vi "Line Configuration Dialog.vi"(8 "error in":errorcluster, 9 "engine configuration in":refnum<class "engine configuration.lvclass">, 10 "tag bus configurable plugin module configuration":refnum<class "Sequencer Module configuration.lvclass">, 11 "Line":T3) -> (0 "error out":errorcluster, 1 "success":bool, 2 "changed":bool, 3 "Mappings out":T2)   [LabVIEW 2015, in "Sequencer Module editor node.lvclass"]
doc: "A dialog for allowing a user to specify the values of a new line."
uses:
  Sequencer Module editor node.lvclass
  module/configuration/Line.ctl
  <vilib>/NI/Tag Bus Module Framework/channel/TBM channel.lvclass
  classes/Sequence/Config/Sequence Config.lvclass
  Mappings.ctl
  Map.ctl
  module/configuration/permissions.ctl
  <vilib>/NI/Module Execution Interface/Engine Configuration/engine configuration.lvclass
  module/configuration/Sequencer Module configuration.lvclass
  <vilib>/NI/Configuration Framework/serializable configuration/NISE_CEF_serializable configuration.lvclass/NISE_CEF_serializable configuration.ctl
  <vilib>/NI/Configuration Framework/serializable configuration/Read UID.vi
  <vilib>/Utility/LVClass/Get LV Class Name.vi
  <vilib>/NI/Configuration Framework/error generator/NISE_error generator.vi
  <vilib>/NI/Tag Bus/tag/tag descriptor.lvclass
  <vilib>/NI/DCAF UI Toolkit/Controls/DCAF UI Elements.lvlib
panel:
  out "errors":string
  in  "Access Type":T1
  in  "Tag":i32(listbox)
  in  "Data Type":i32(listbox)
  in  "Channel Name":string
  in  "cancel":bool
  in  "ok":bool
  # "#CodeRecommended Add implementation details here. For example, a shared variable URL."
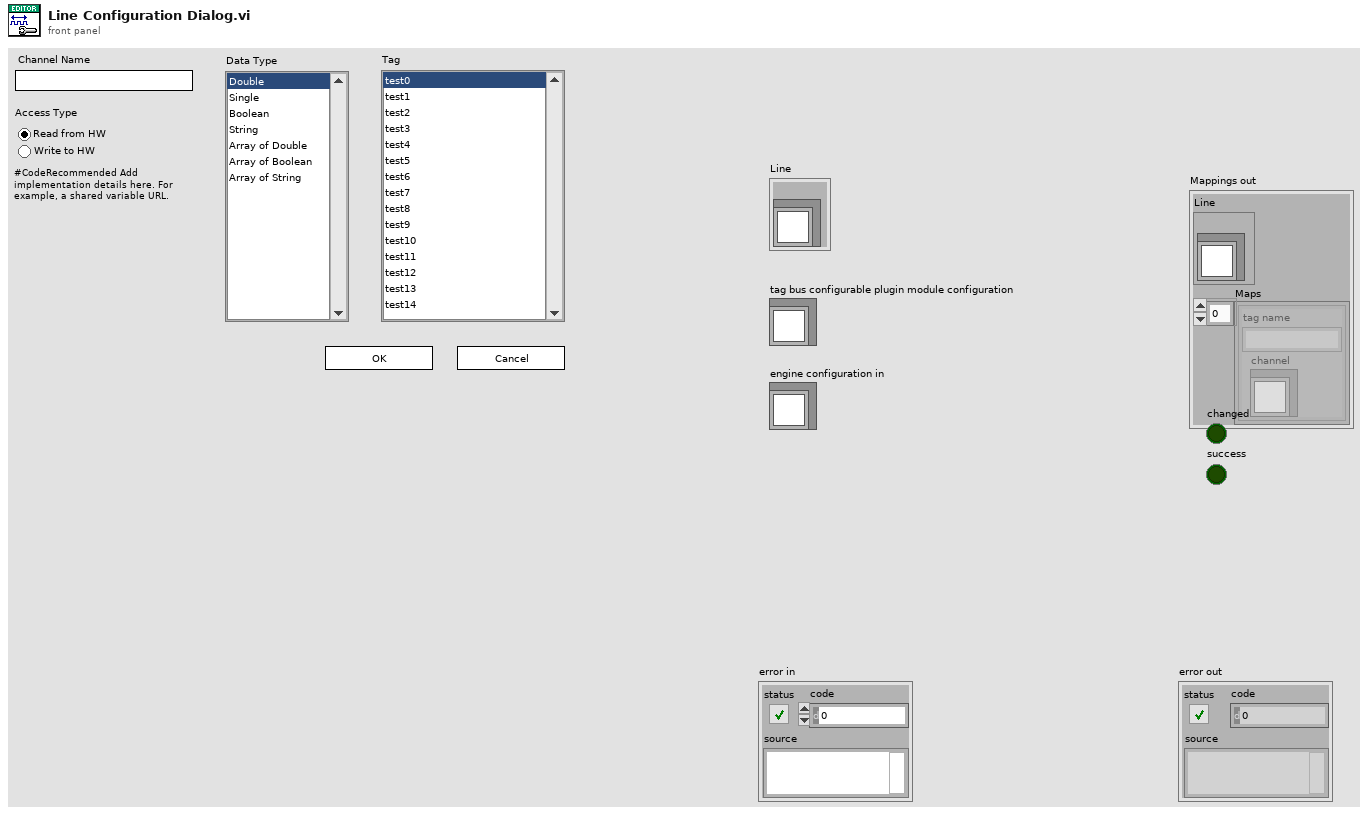
[diagram p1: front panel]
types:
  T1 = typedef "Sequencer Module configuration.lvclass/permissions.ctl" = enum32{"Read from HW", "Write to HW"}
  T2 = typedef "Sequencer Module editor node.lvclass/Mappings.ctl" = cluster{"Line":T3, "Maps":T4[]}
  T3 = typedef "Sequencer Module configuration.lvclass/Line.ctl" = cluster{"Sequence":refnum<class "Sequence Config.lvclass">}
  T4 = typedef "Sequencer Module editor node.lvclass/Map.ctl" = cluster{"channel":refnum<class "TBM channel.lvclass">, "tag name":string}
  T5 = typedef "tag bus.lvlib/tag descriptor.lvclass/Data Type.ctl" = enum16{"Double", "Single", "I64", "I32", "I16", "I8", "U64", "U32", "U16", "U8", "Boolean", "String", "Array of Double", "Array of Single", "Array of I64", "Array of I32", "Array of I16", "Array of I8", "Array of U64", "Array of U32", "Array of U16", "Array of U8", "Array of Boolean", "Array of String"}
  T6 = typedef "TBM channel.lvclass/channel classification.ctl" = enum16{"input data", "output data", "processing parameter", "processing result"}
  T7 = enum8{"Enabled", "Disabled", "Disabled and Grayed Out"}
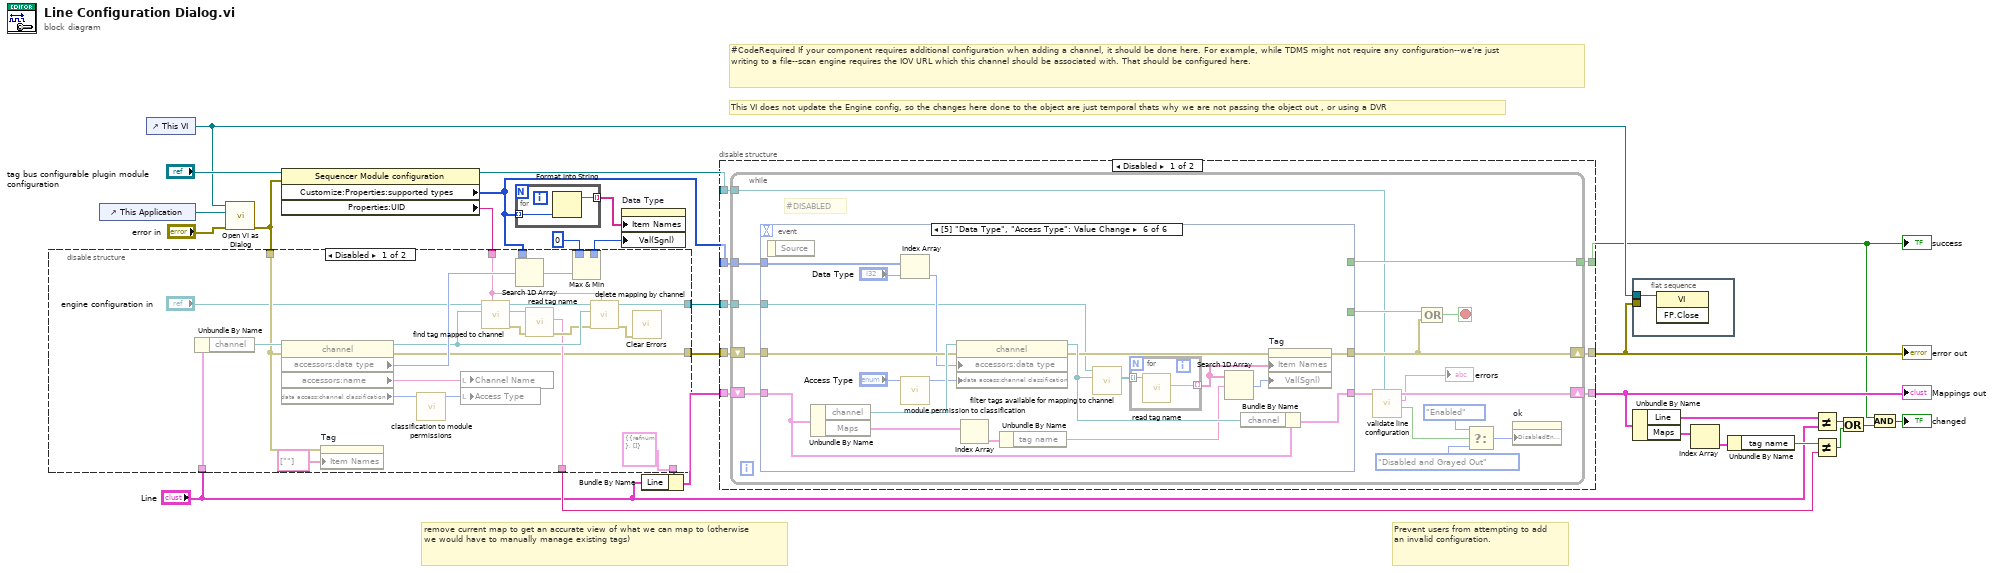
[diagram p0: block diagram]
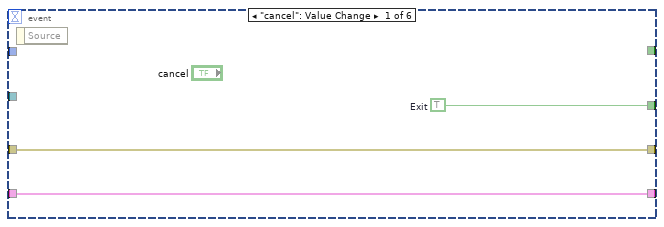
[diagram p3: hidden frame]
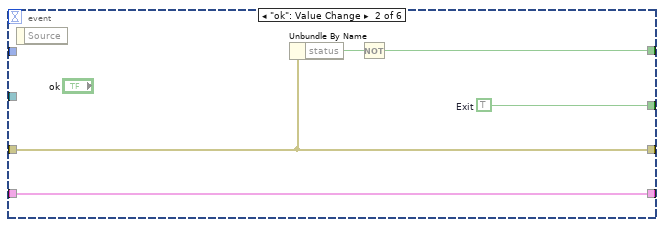
[diagram p4: hidden frame]
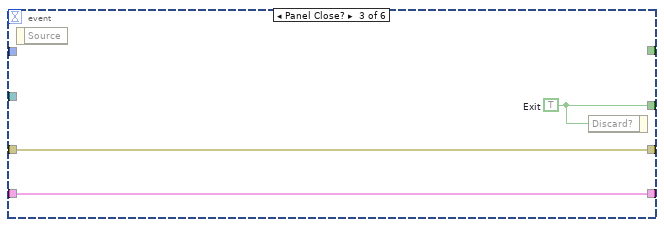
[diagram p5: hidden frame]
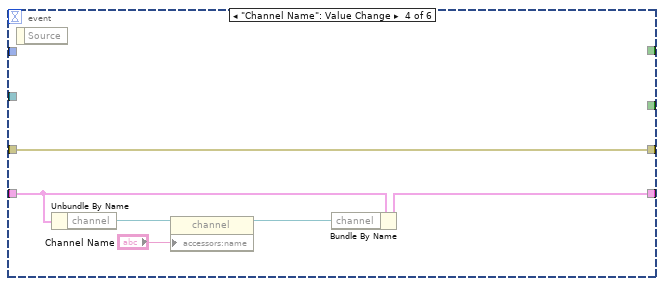
[diagram p6: hidden frame]
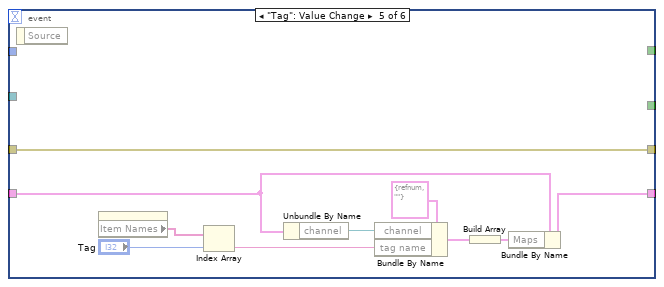
[diagram p7: hidden frame]
diagram:
  # "Prevent users from attempting to add an invalid configuration."
  # "This VI does not update the Engine config, so the changes here done to the object are just temporal thats why we are not passing the object out , or using a DVR"
  # "remove current map to get an accurate view of what we can map to (otherwise we would have to manually manage existing tags)"
  # "#CodeRequired If your component requires additional configuration when adding a channel, it should be done here. For example, while TDMS might not require any configuration--we're just writing to a file--scan engine requires the IOV URL which this channel should be associated with. That should be configured here."
  n1 = control-ref of="This Application"() -> (w21:refnum<vi>)
  n2 = control-ref of="This VI"() -> (w11:refnum<vi>)
  n3 = call <vilib>:"Open VI as Dialog.vi"("error in (no error)"="error in", "This Application"=w21, "VI in"=w11) -> ("error out"=w19:errorcluster)  [unwired: 8 in]
  n4 = property class="Sequencer Module configuration"(reference="tag bus configurable plugin module configuration", error in=w19) -> (reference out=w18:refnum<class "Sequencer Module configuration.lvclass">, "Customize:Properties:supported types"=w1:T5[], "Properties:UID"=w7:string)  [unwired: 1 out]
  n5 = disable-structure shown="Disabled" {
    disable-tunnel: [w52 _] -> w28
    disable-tunnel: [T2 {"Line"={"Sequence"=refnum}, "Maps"=[]} ("Mappings out") _] -> w25
    disable-tunnel: w19 -> [w46 _]
    disable-tunnel: 0 ("f") -> [w41 _]
    disable-tunnel: [w37 _] -> w10
    disable-tunnel: "Line" -> [w36 _]
    disable-tunnel: [w35 _] -> w8
    disable-tunnel: w7 -> [w33 _]
    disable-tunnel: [w31 _] -> w6
    disable-tunnel: w1 -> [w29 _]
    frame Disabled {
      n6 = Unbundle By Name(w36) -> ("channel"=w51:refnum<class "TBM channel.lvclass">)
      n7 = property class="channel"(reference=w51, error in=w46) -> (reference out=w43:refnum<class "TBM channel.lvclass">, error out=w31:errorcluster, "accessors:data type"=w49:T5, "accessors:name"=w30:string, "data access:channel classification"=w32:T6)
      n8 = property on="Tag" class="LstBox (strict)"(error in=w46, "Item Names"=string[] [""]) -> ()  [unwired: 1 in, 2 out]
      n9 = call "classification to module permissions.vi"("channel classification"=w32) -> ("permissions"=w34:T1)  [unwired: 10 in]
      n10 = local write "Channel Name"(w30) -> ()
      n11 = local write "Access Type"(w34) -> ()
      n12 = call <vilib>:"find tag mapped to channel.vi"("owner"=w33, "channel"=w43, "engine configuration in"="engine configuration in") -> ("error out"=w39:errorcluster, "tag"=w40:refnum<class "tag descriptor.lvclass">, "engine configuration out"=w44:refnum<class "engine configuration.lvclass">)  [unwired: 6 in]
      n13 = Search 1D Array(1D array=w29, element=w49) -> (index of element=w42:i32)  [unwired: 1 in]
      n14 = call <vilib>:"read tag name.vi"("error in"=w39, "system tag in"=w40) -> ("error out"=w38:errorcluster, "name"=w37:string)  [unwired: 7 in, 1 out]
      n15 = Max & Min(x=w41, y=w42) -> (max(x,y)=w35:i32)  [unwired: 1 out]
      n16 = call <vilib>:"delete mapping by channel.vi"("owner ID"=w33, "error in"=w38, "channel"=w43, "engine configuration in"=w44) -> ("error out"=w48:errorcluster, "engine configuration out"=w52:refnum<class "engine configuration.lvclass">)  [unwired: 6 in]
      n17 = call <vilib>:"Clear Errors.vi"("error in (no error)"=w48) -> ()  [unwired: 5 in, 2 out]
    }
    frame Enabled {
    }
  }
  n18 = for {
    tunnel: w1 -> [w54] mode=indexing
    tunnel: [w53] -> w27 mode=indexing
    n19 = Format Into String(w54) -> (resulting string=w53:string)  [unwired: 3 in, 1 out]
  }
  n20 = property on="Data Type" class="LstBox (strict)"("Item Names"=w27, "Val(Sgnl)"=w8) -> ()  [unwired: 2 in, 2 out]
  n21 = Bundle By Name(cluster=w25, "Line"="Line") -> (w24:T2)
  n22 = disable-structure shown="Disabled" {
    disable-tunnel: w28 -> [w62 _]
    disable-tunnel: w24 -> [w61 _]
    disable-tunnel: [w60 _] -> w22
    disable-tunnel: w18 -> [w59 _]
    disable-tunnel: w6 -> [w58 _]
    disable-tunnel: [w57 _] -> w5
    disable-tunnel: [w56 _] -> w4
    disable-tunnel: w1 -> [w55 _]
    frame Disabled {
      n23 = while {
        shift-right: [w70] -> w57
        shift-left: w58 -> [w77]
        tunnel: [w76] -> w56
        shift-right: [w71] -> w60
        shift-left: w61 -> [w73]
        tunnel: w62 -> [w78]
        tunnel: w59 -> [w63]
        tunnel: w55 -> [w65]
        stop <- w74 stop-if-true
        # "#DISABLED"
        n24 = event shown="[5] \"Data Type\", \"Access Type\": Value Change" {
          selector: _ -> [_ _ _ _ _ _]
          dyn-events: _ -> [_ _ _ _ _ _]
          timeout: _ -> [_ _ _ _ _ _]
          tunnel: w78 -> [_ _ _ _ _ w106]
          tunnel: w77 -> [w81 w84 w89 w95 w105 w118]
          tunnel: [w81 w84 w89 w95 w105 w113] -> w70
          tunnel: [_ w82 _ _ _ _] -> w76
          tunnel: [w79 w85 w87 _ _ _] -> w75
          tunnel: w73 -> [w80 w86 w88 w93 w96 w107]
          tunnel: [w80 w86 w88 w94 w98 w121] -> w72
          tunnel: w65 -> [_ _ _ _ _ w117]
          event "cancel": Value Change {
            w79 = TRUE  # Exit
            n25 = event-data() -> ()  [unwired: 1 in, 1 out]
          }
          event "ok": Value Change {
            w85 = TRUE  # Exit
            n26 = event-data() -> ()  [unwired: 1 in, 1 out]
            n27 = Unbundle By Name(w84) -> ("status"=w83:bool)
            n28 = Not(x=w83) -> (.not. x?=w82:bool)
          }
          event Panel Close? {
            w87 = TRUE  # Exit
            n29 = event-data() -> ()  [unwired: 1 in, 1 out]
            n30 = event-data("Discard?"=w87) -> ()  [unwired: 1 in, 1 out]
          }
          event "Channel Name": Value Change {
            n31 = event-data() -> ()  [unwired: 1 in, 1 out]
            n32 = Unbundle By Name(w93) -> ("channel"=w92:refnum<class "TBM channel.lvclass">)
            n33 = property class="channel"(reference=w92, "accessors:name"="Channel Name") -> (reference out=w91:refnum<class "TBM channel.lvclass">)  [unwired: 1 in, 1 out]
            n34 = Bundle By Name(cluster=w93, "channel"=w91) -> (w94:T2)
          }
          event "Tag": Value Change {
            n35 = event-data() -> ()  [unwired: 1 in, 1 out]
            n36 = property on="Tag" class="LstBox (strict)"() -> ("Item Names"=w103:string[])  [unwired: 2 in, 2 out]
            n37 = Index Array(array=w103, index="Tag") -> (element=w97:string)
            n38 = Unbundle By Name(w96) -> ("channel"=w101:refnum<class "TBM channel.lvclass">)
            n39 = Bundle By Name(cluster=T4 {"channel"=refnum, "tag name"=""} ("Map"), "channel"=w101, "tag name"=w97) -> (w100:T4)
            n40 = Build Array(w100) -> (w99:T4[])
            n41 = Bundle By Name(cluster=w96, "Maps"=w99) -> (w98:T2)
          }
          event "Data Type": Value Change {
            n42 = event-data() -> ()  [unwired: 1 in, 1 out]
            n43 = Unbundle By Name(w107) -> ("channel"=w124:refnum<class "TBM channel.lvclass">, "Maps"=w108:T4[])
            n44 = Index Array(array=w117, index="Data Type") -> (element=w115:T5)
            n45 = call "module permission to classification.vi"("display permissions"="Access Type") -> ("channel classification"=w123:T6)  [unwired: 10 in]
            n46 = property class="channel"(reference=w124, error in=w118, "accessors:data type"=w115, "data access:channel classification"=w123) -> (reference out=w122:refnum<class "TBM channel.lvclass">, error out=w114:errorcluster)
            n47 = Index Array(array=w108) -> (element=w110:T4)  [unwired: 1 in]
            n48 = Unbundle By Name(w110) -> ("tag name"=w109:string)
            n49 = call-dynamic "filter tags available for mapping to channel.vi"("channel to map to"=w122, "engine configuration in"=w106) -> ("filtered tags"=w120:refnum<class "tag descriptor.lvclass">[])  [unwired: 8 in, 1 out]
            n50 = for {
              tunnel: w120 -> [w126] mode=indexing
              tunnel: [w125] -> w112 mode=indexing
              n51 = call <vilib>:"read tag name.vi"("system tag in"=w126) -> ("name"=w125:string)  [unwired: 8 in, 2 out]
            }
            n52 = Search 1D Array(1D array=w112, element=w109) -> (index of element=w111:i32)  [unwired: 1 in]
            n53 = Bundle By Name(cluster=w107, "channel"=w122) -> (w121:T2)
            n54 = property on="Tag" class="LstBox (strict)"(error in=w114, "Item Names"=w112, "Val(Sgnl)"=w111) -> (error out=w113:errorcluster)  [unwired: 1 in, 1 out]
          }
        }
        n55 = call "validate line configuration.vi"("Module Config"=w63, "Mappings in"=w72) -> ("valid?"=w69:bool, "errors"=→"errors":string, "Mappings out"=w71:T2)  [unwired: 7 in]
        n56 = Compound Arithmetic op=OR(w75, w70) -> (w74:bool)
        n57 = Select(t=T7."Enabled" ("Disabled"), s=w69, f=T7."Disabled and Grayed Out") -> (s? t:f=w66:T7)
        n58 = property on="ok" class="Bool"("DisabledEnum"=w66) -> ()  [unwired: 2 in, 2 out]
      }
    }
    frame Enabled {
    }
  }
  "error out" <- w5
  "success" <- w4
  "Mappings out" <- w22
  n59 = flat-sequence {
    tunnel: w5 -> [_]
    tunnel: w11 -> [w127]
    frame #0 {
      n60 = invoke class="VI" method="FP.Close"(reference=w127) -> ()  [unwired: 2 in, 3 out]
    }
  }
  n61 = Unbundle By Name(w22) -> ("Line"=w23:T3, "Maps"=w16:T4[])
  n62 = Index Array(array=w16) -> (element=w15:T4)  [unwired: 1 in]
  n63 = Unbundle By Name(w15) -> ("tag name"=w14:string)
  n64 = Not Equal?(x=w23, y="Line") -> (x != y?=w12:bool)
  n65 = Not Equal?(x=w14, y=w10) -> (x != y?=w13:bool)
  n66 = Or(x=w12, y=w13) -> (x .or. y?=w3:bool)
  n67 = And(x=w4, y=w3) -> (x .and. y?=→"changed":bool)
